vi "monitor get expected sync delta raw.vi"(11 "output_rate_hz":u32) -> (3 "function return":u32)   [LabVIEW 2019, in "apdm.lvlib"]
doc: "APDM_EXPORT uint32_t apdm_monitor_get_expected_sync_delta_raw(const uint32_t output_rate_hz);"
uses:
  apdm.lvlib
  Lee Lab/CP FES Walking 2018/Code/Working/LabVIEW/apdm.dll
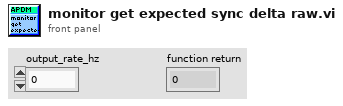
[diagram p1: front panel]
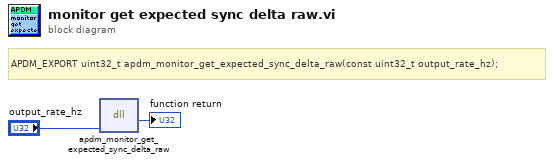
[diagram p0: block diagram]
diagram:
  # "APDM_EXPORT uint32_t apdm_monitor_get_expected_sync_delta_raw(const uint32_t output_rate_hz);"
  n1 = dll-call lib="C:/Users/jfalesi/Dropbox/Lee Lab/CP FES Walking 2018/Code/Working/LabVIEW/apdm.*" fn="apdm_monitor_get_expected_sync_delta_raw"("output_rate_hz"="output_rate_hz") -> (→"function return":u32)  [unwired: 4 in, 2 out]
